vi "main_PC.vi"() -> ()   [LabVIEW 2017]
panel:
  in  "Tab Control":enum32{"Page 1", "Page 2"}(tab)
  in  "Menu Ring":u16(ring) items=["OFF", "Automatic", "Manual"]
  out "Waveform Chart":T1(graph) caption="Response Chart"
  in  "Pause Button":bool
  in  "Reset Chart":bool
  in  "Save as Excel":bool
  in  "Save as image":bool
  in  "Block Diagram":bool
  out "P":dbl
  out "Control Action":bool
  in  "Pressure setpoint":dbl=7.0 min=1.5 max=7.0
  in  "Comperssor":bool=TRUE
  in  "ON/OFF":bool
  in  "Exit":bool
  out "NI1":tag caption="NI device"
  in  "P 2":dbl
  in  "Main board":bool
  # "Pressure Control Training System"
  # "( 1.5-7 ) bar"
  # "Pressure sensor Reading"
  # "bar"
  # "Block Diagram of \nthe Pressure Closed-loop Control System"
  # "ON/OFF"
  # "Automatic mode"
  # "Actuator ON/OFF"
  # "desired P"
  # "Controller\n(ON/OFF)"
  # "Actuator\n(Compressor)"
  # "System"
  # "Pressure diff."
  # "error signal"
  # "+"
  # "-"
  # "Control Action\n(0 - 1)"
  # "actual P"
  # "Pressure sensor"
  # "Block Diagram of \nthe Pressure Open-loop Control System"
  # "Actuator ON/OFF"
  # "Actuator\n(Compressor)"
  # "Pressure diff."
  # "System"
  # "Press"
  # "Bush Button"
  # "Control Action\n(0 - 1)"
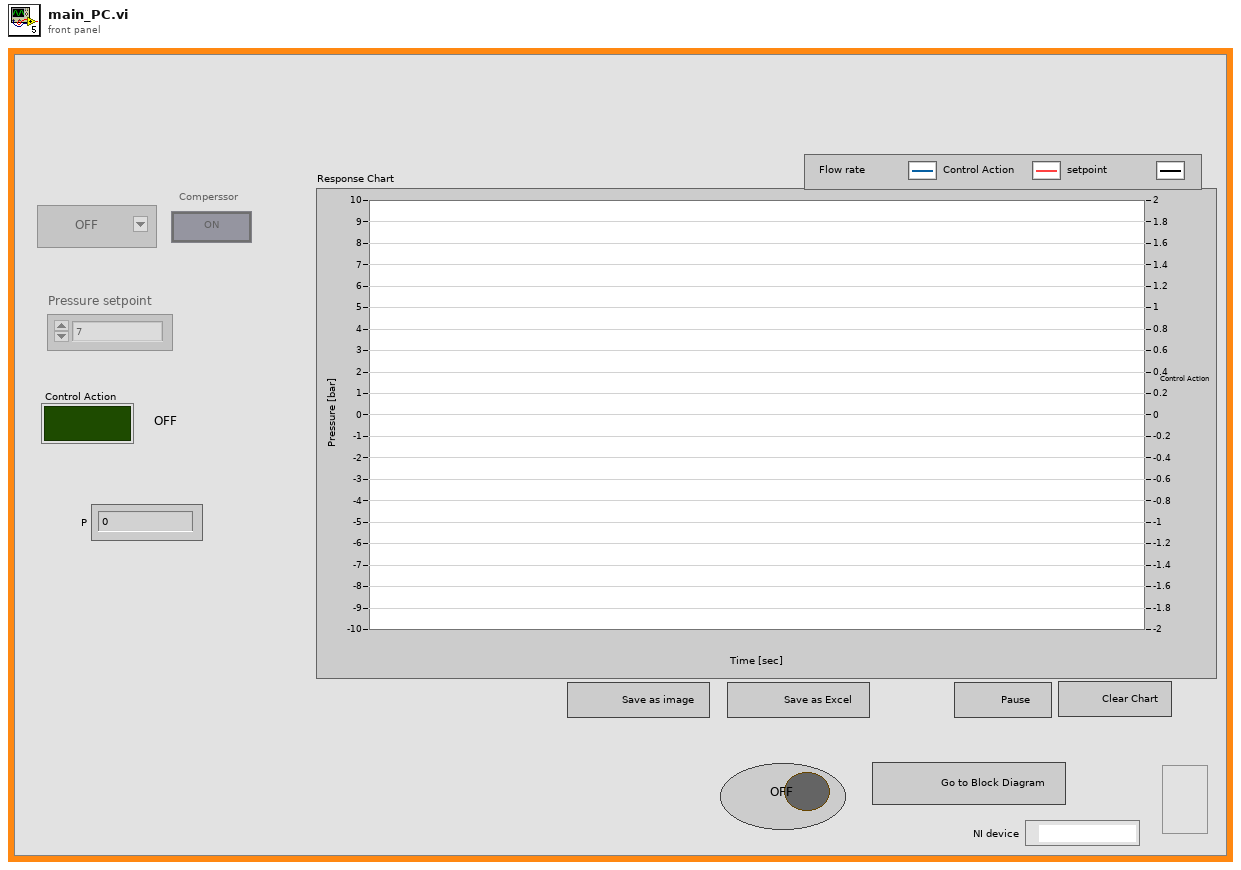
[diagram p1: front panel]
types:
  T1 = cluster{"Scalar":dbl, "f":dbl, "Flow rate setpoint":dbl}
  T2 = enum32{"Invalid", "Standard", "Closed", "Hidden", "Minimized", "Maximized"}
  T3 = enum8{"Enabled", "Disabled", "Disabled and Grayed Out"}
  T4 = cluster{"Scalar":dbl, "f":dbl, "Flow rate setpoint":dbl}[]
  T5 = cluster{"Scalar":dbl, i16, "Pressure setpoint":dbl}
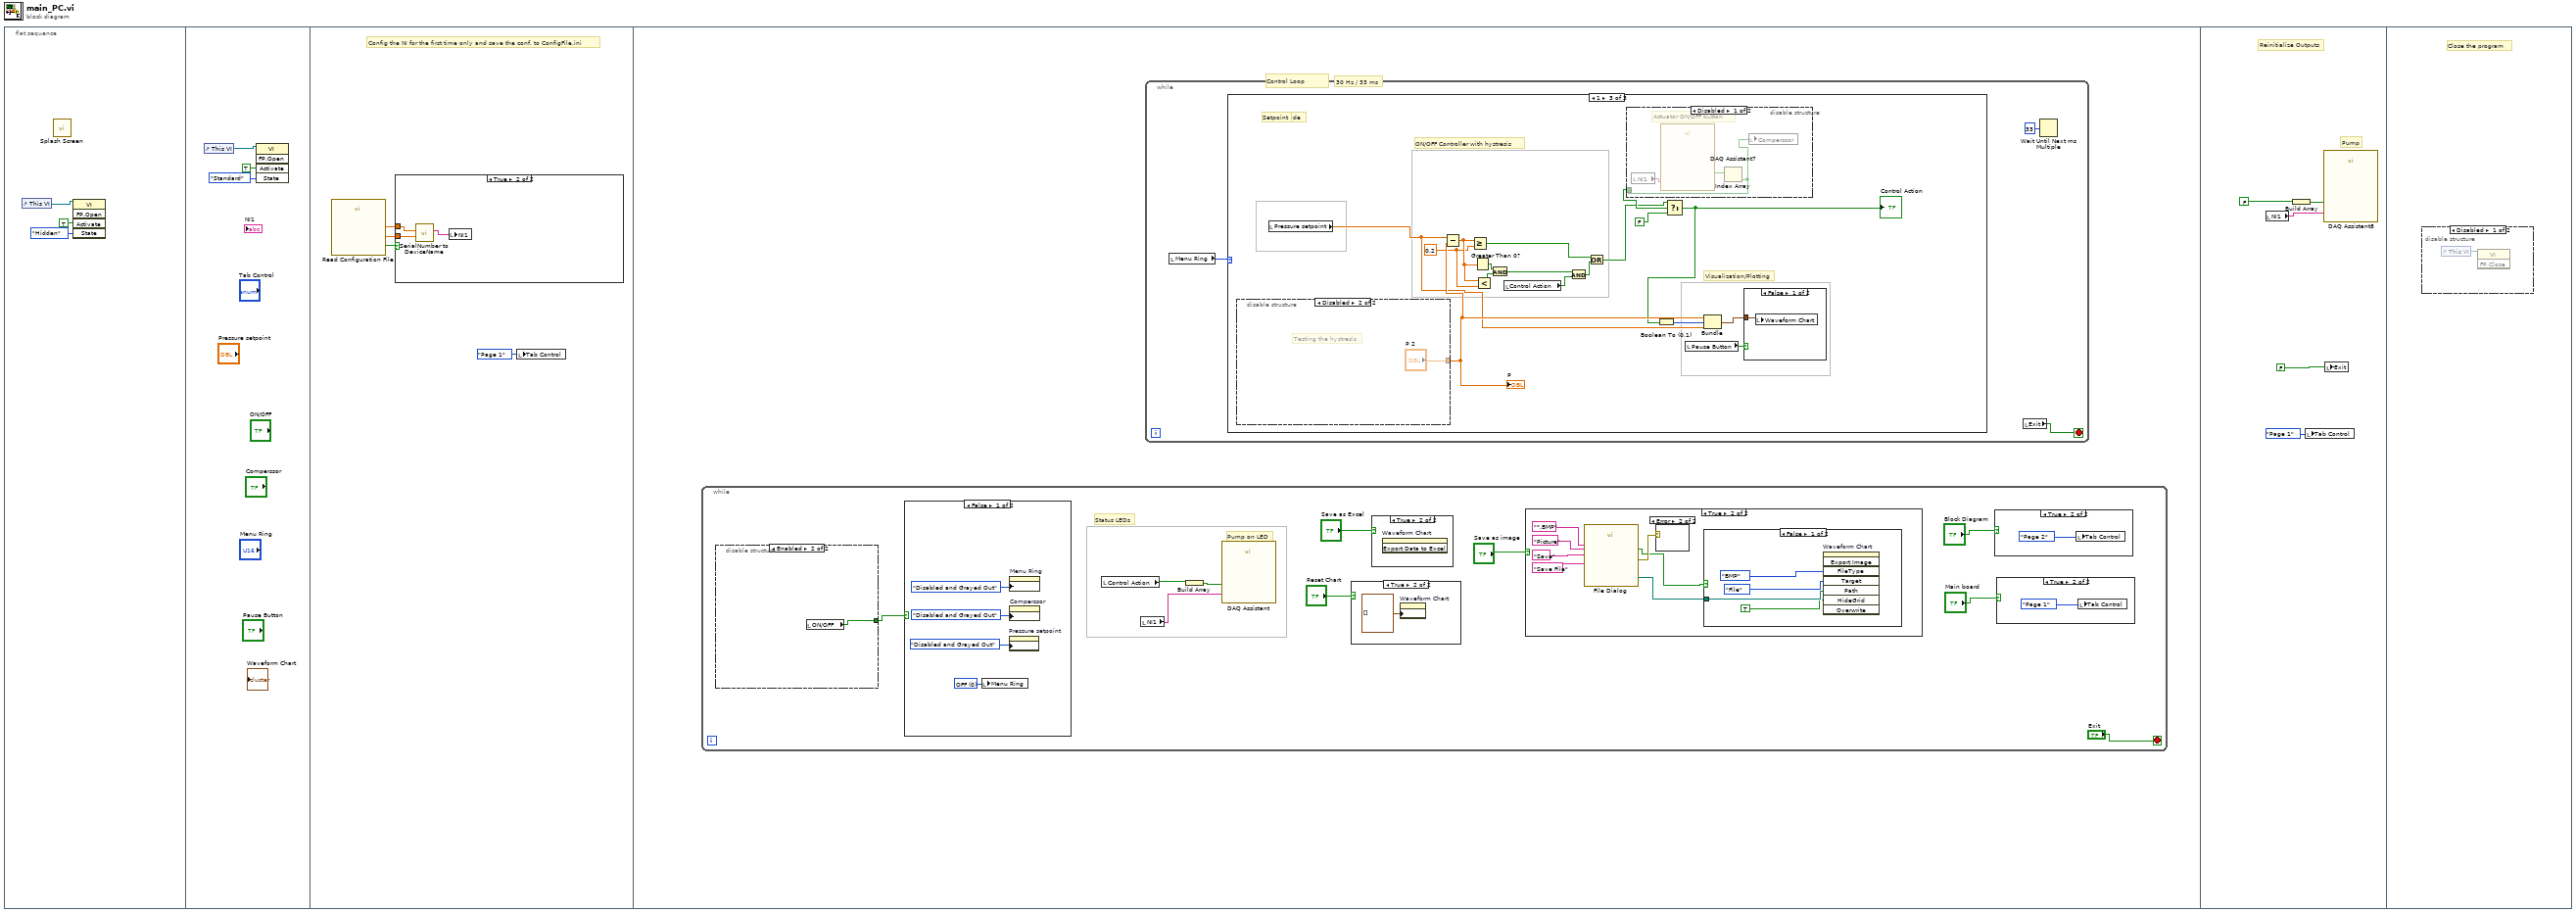
[diagram p0: block diagram]
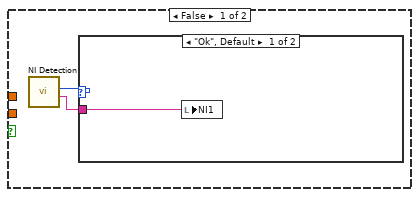
[diagram p2: hidden frame]
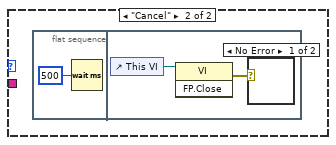
[diagram p3: hidden frame]
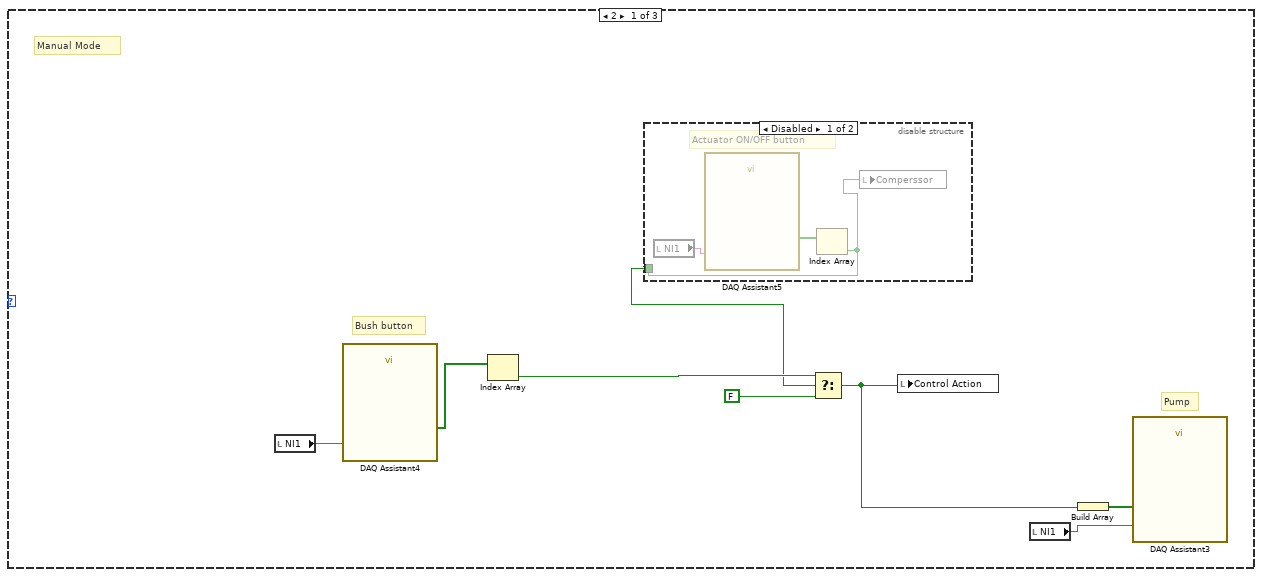
[diagram p5: hidden frame]
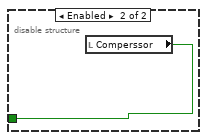
[diagram p6: hidden frame]
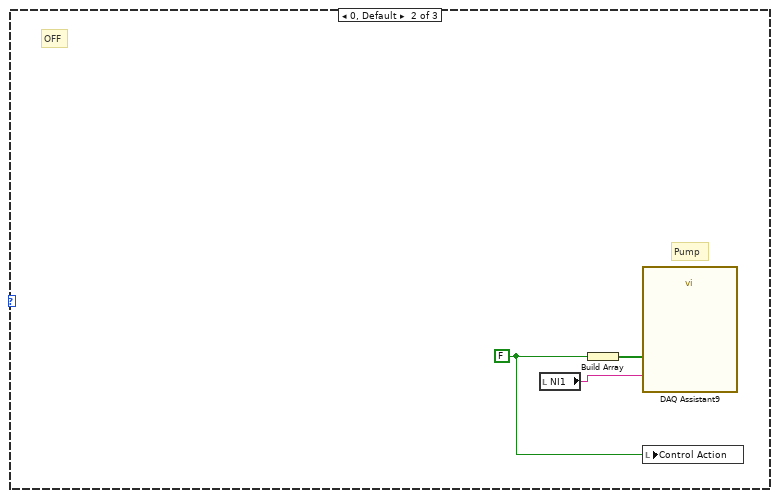
[diagram p7: hidden frame]
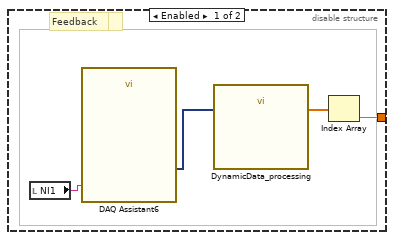
[diagram p8: hidden frame]
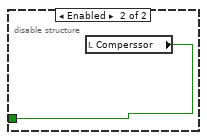
[diagram p9: hidden frame]
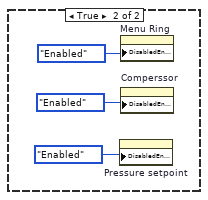
[diagram p11: hidden frame]
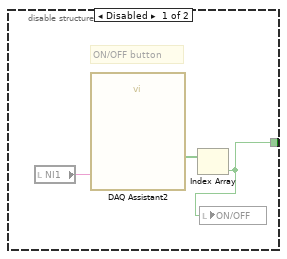
[diagram p12: hidden frame]
diagram:
  n1 = flat-sequence {
    frame #0 {
      n2 = control-ref of="This VI"() -> (w3:refnum<vi>)
      n3 = call "Splash Screen.vi"() -> ()  [unwired: 11 in, 1 out]
      n4 = invoke class="VI" method="FP.Open"(reference=w3, "Activate"=TRUE ("Activate?"), "State"=T2."Hidden") -> ()  [unwired: 2 in, 5 out]
    }
    frame #1 {
      n5 = control-ref of="This VI"() -> (w4:refnum<vi>)
      n6 = invoke class="VI" method="FP.Open"(reference=w4, "Activate"=TRUE ("Activate?"), "State"=T2."Standard") -> ()  [unwired: 2 in, 5 out]
    }
    frame #2 {
      # "Config the NI for the first time only and save the conf. to ConfigFile.ini"
      n7 = call "Read Configuration File.vi"() -> ("Serial Numbers Found"=w8:bool, "NI1"=w9:dbl, "NI2"=w10:dbl)  [unwired: 13 in]
      n8 = case shown="True" w8 {
        tunnel: w9 -> [_ w19]
        tunnel: w10 -> [_ w18]
        frame False {
          n9 = call "NI Detection.vi"() -> ("NI 1"=w11:tag, "Ok/Cancel"=w12:enum16{"Ok", "Cancel"})  [unwired: 8 in, 1 out]
          n10 = case shown="\"Ok\", Default" w12 {
            tunnel: w11 -> [w13 _]
            frame "Ok", Default {
              n11 = local write "NI1"(w13) -> ()
            }
            frame "Cancel" {
              n12 = flat-sequence {
                frame #0 {
                  n13 = Wait (ms)(milliseconds to wait=u32 500) -> ()  [unwired: 1 out]
                }
                frame #1 {
                  n14 = control-ref of="This VI"() -> (w16:refnum<vi>)
                  n15 = invoke class="VI" method="FP.Close"(reference=w16) -> (error out=w15:errorcluster)  [unwired: 2 in, 2 out]
                  n16 = case shown="No Error" w15 {
                    frame No Error {
                    }
                    frame Error {
                    }
                  }
                }
              }
            }
          }
        }
        frame True {
          n17 = call "SerialNumber to DeviceName.vi"("NI2 Serial Number"=w18, "NI1 Serial Number"=w19) -> ("NI1 Device Name"=w17:tag)  [unwired: 8 in, 1 out]
          n18 = local write "NI1"(w17) -> ()
        }
      }
      n19 = local write "Tab Control"(enum32{"Page 1", "Page 2"}."Page 1" ("Tab Control")) -> ()
    }
    frame #3 {
      # "30 Hz / 33 ms"
      # "Control Loop"
      n20 = while {
        stop <- "Exit" stop-if-true
        # "Pump on LED"
        # "Status LEDs"
        n21 = disable-structure shown="Enabled" {
          disable-tunnel: [w82 w85] -> w65
          frame Disabled {
            # "ON/OFF button"
            n22 = local read "NI1"() -> (w84:tag)
            n23 = call "DAQ Assistant2"("device name"=w84) -> ("data"=w83:bool[])  [unwired: 16 in, 2 out]
            n24 = Index Array(array=w83) -> (element=w82:bool)  [unwired: 1 in]
            n25 = local write "ON/OFF"(w82) -> ()
          }
          frame Enabled {
            n26 = local read "ON/OFF"() -> (w85:bool)
          }
        }
        n27 = case shown="False" w65 {
          frame False {
            w75 = u16 0 items=["OFF", "Automatic", "Manual"] ("Menu Ring")
            n28 = local write "Menu Ring"(w75) -> ()
            n29 = property on="Pressure setpoint" class="DigNum (strict)"("DisabledEnum"=T3."Disabled and Grayed Out" ("Disabled")) -> ()  [unwired: 2 in, 2 out]
            n30 = property on="Menu Ring" class="Ring (strict)"("DisabledEnum"=T3."Disabled and Grayed Out" ("Disabled")) -> ()  [unwired: 2 in, 2 out]
            n31 = property on="Comperssor" class="Bool (strict)"("DisabledEnum"=T3."Disabled and Grayed Out" ("Disabled")) -> ()  [unwired: 2 in, 2 out]
          }
          frame True {
            n32 = property on="Pressure setpoint" class="DigNum (strict)"("DisabledEnum"=T3."Enabled" ("Disabled")) -> ()  [unwired: 2 in, 2 out]
            n33 = property on="Menu Ring" class="Ring (strict)"("DisabledEnum"=T3."Enabled" ("Disabled")) -> ()  [unwired: 2 in, 2 out]
            n34 = property on="Comperssor" class="Bool (strict)"("DisabledEnum"=T3."Enabled" ("Disabled")) -> ()  [unwired: 2 in, 2 out]
          }
        }
        n35 = local read "Control Action"() -> (w67:bool)
        n36 = local read "NI1"() -> (w69:tag)
        n37 = Build Array(w67) -> (w68:bool[])
        n38 = call "DAQ Assistant"("data"=w68, "device name"=w69) -> ()  [unwired: 16 in, 2 out]
        n39 = case shown="True" "Reset Chart" {
          frame False {
          }
          frame True {
            n40 = property on="Waveform Chart" class="WFChart (strict)"("History Data"=T4 []) -> ()  [unwired: 2 in, 2 out]
          }
        }
        n41 = case shown="True" "Save as Excel" {
          frame False {
          }
          frame True {
            n42 = invoke on="Waveform Chart" class="WFChart (strict)" method="Export Data to Excel"() -> ()  [unwired: 3 in, 3 out]
          }
        }
        n43 = case shown="True" "Save as image" {
          frame False {
          }
          frame True {
            n44 = call "File Dialog"("prompt"="Save File", "button label"="Save", "pattern (all files)"="*.BMP", "pattern label"="Picture") -> ("selected path"=w87:path, "cancelled"=w86:bool, "error out"=w88:errorcluster)  [unwired: 8 in, 1 out]
            n45 = case shown="Error" w88 {
              frame No Error {
              }
              frame Error {
              }
            }
            n46 = case shown="False" w86 {
              tunnel: w87 -> [w94 _]
              frame False {
                n47 = invoke on="Waveform Chart" class="WFChart (strict)" method="Export Image"("FileType"=enum32{"BMP", "EPS", "EMF", "PICT"}."BMP" ("File Type"), "Target"=enum32{"File", "Clipboard"}."File", "Path"=w94, "HideGrid"=TRUE ("Hide Grid")) -> ()  [unwired: 4 in, 8 out]
              }
              frame True {
              }
            }
          }
        }
        n48 = case shown="True" "Block Diagram" {
          frame False {
          }
          frame True {
            n49 = local write "Tab Control"(enum32{"Page 1", "Page 2"}."Page 2" ("Tab Control")) -> ()
          }
        }
        n50 = case shown="True" "Main board" {
          frame False {
          }
          frame True {
            n51 = local write "Tab Control"(enum32{"Page 1", "Page 2"}."Page 1" ("Tab Control")) -> ()
          }
        }
      }
      n52 = while {
        stop <- w20 stop-if-true
        n53 = local read "Menu Ring"() -> (w21:u16)
        n54 = case shown="1" w21 {
          frame 2 {
            # "Pump"
            # "Manual Mode"
            # "Bush button"
            n55 = local read "NI1"() -> (w28:tag)
            n56 = call "DAQ Assistant4"("device name"=w28) -> ("data"=w27:bool[])  [unwired: 16 in, 2 out]
            n57 = Index Array(array=w27) -> (element=w30:bool)  [unwired: 1 in]
            n58 = disable-structure shown="Disabled" {
              disable-tunnel: [w32 w34] -> w29
              frame Disabled {
                # "Actuator ON/OFF button"
                n59 = local read "NI1"() -> (w31:tag)
                n60 = call "DAQ Assistant5"("device name"=w31) -> ("data"=w33:bool[])  [unwired: 16 in, 2 out]
                n61 = Index Array(array=w33) -> (element=w32:bool)  [unwired: 1 in]
                n62 = local write "Comperssor"(w32) -> ()
              }
              frame Enabled {
                n63 = local read "Comperssor"() -> (w34:bool)
              }
            }
            n64 = Select(t=w30, s=w29, f=FALSE) -> (s? t:f=w23:bool)
            n65 = local write "Control Action"(w23) -> ()
            n66 = local read "NI1"() -> (w24:tag)
            n67 = Build Array(w23) -> (w25:bool[])
            n68 = call "DAQ Assistant3"("data"=w25, "device name"=w24) -> ()  [unwired: 16 in, 2 out]
          }
          frame 0, Default {
            w35 = FALSE
            # "OFF"
            # "Pump"
            n69 = local read "NI1"() -> (w36:tag)
            n70 = Build Array(w35) -> (w37:bool[])
            n71 = call "DAQ Assistant9"("data"=w37, "device name"=w36) -> ()  [unwired: 16 in, 2 out]
            n72 = local write "Control Action"(w35) -> ()
          }
          frame 1 {
            w45 = 0.2 ("y")
            # "AUTO mode"
            # "Setpoint"
            # "Visualization/Plotting"
            # "ON/OFF Controller with hystresis"
            n73 = disable-structure shown="Disabled" {
              disable-tunnel: [w55 "P 2"] -> w51
              frame Enabled {
                # "Feedback"
                # "Flow sensor"
                n74 = local read "NI1"() -> (w56:tag)
                n75 = call "DAQ Assistant6"("device name"=w56) -> ("data"=w58:dynamicdata)  [unwired: 16 in, 2 out]
                n76 = call "DynamicData_processing.vi"("data"=w58) -> ("DATA"=w57:dbl[])
                n77 = Index Array(array=w57) -> (element=w55:dbl)  [unwired: 1 in]
              }
              frame Disabled {
                # "Testing the hystresis"
              }
            }
            "P" <- w51
            n78 = local read "Pressure setpoint"() -> (w38:dbl)
            n79 = Subtract(x=w38, y=w51) -> (x-y=w46:dbl)
            n80 = Greater Or Equal?(x=w46, y=w45) -> (x >= y?=w49:bool)
            n81 = Greater Than 0?(x=w46) -> (x > 0?=w48:bool)
            n82 = Less?(x=w46, y=w45) -> (x < y?=w47:bool)
            n83 = And(x=w48, y=w47) -> (x .and. y?=w44:bool)
            n84 = local read "Control Action"() -> (w43:bool)
            n85 = And(x=w44, y=w43) -> (x .and. y?=w42:bool)
            n86 = Or(x=w49, y=w42) -> (x .or. y?=w41:bool)
            n87 = disable-structure shown="Disabled" {
              disable-tunnel: [w61 w63] -> w53
              frame Disabled {
                # "Actuator ON/OFF button"
                n88 = local read "NI1"() -> (w60:tag)
                n89 = call "DAQ Assistant7"("device name"=w60) -> ("data"=w62:bool[])  [unwired: 16 in, 2 out]
                n90 = Index Array(array=w62) -> (element=w61:bool)  [unwired: 1 in]
                n91 = local write "Comperssor"(w61) -> ()
              }
              frame Enabled {
                n92 = local read "Comperssor"() -> (w63:bool)
              }
            }
            n93 = Select(t=w41, s=w53, f=FALSE) -> (s? t:f=w39:bool)
            "Control Action" <- w39
            n94 = Boolean To (0,1)(Boolean=w39) -> (0, 1=w40:i16)
            n95 = local read "Pause Button"() -> (w52:bool)
            n96 = Bundle("Scalar"=w51, w40, "Pressure setpoint"=w38) -> (w54:T5)  [unwired: 1 in]
            n97 = case shown="False" w52 {
              tunnel: w54 -> [w64 _]
              frame False {
                n98 = local write "Waveform Chart"(w64) -> ()
              }
              frame True {
              }
            }
          }
        }
        n99 = local read "Exit"() -> (w20:bool)
        n100 = Wait Until Next ms Multiple(millisecond multiple=u32 33) -> ()  [unwired: 1 out]
      }
    }
    frame #4 {
      # "Pump"
      # "Reinitialize Outputs"
      n101 = local read "NI1"() -> (w102:tag)
      n102 = Build Array(FALSE) -> (w101:bool[])
      n103 = local write "Tab Control"(enum32{"Page 1", "Page 2"}."Page 1" ("Tab Control")) -> ()
      n104 = call "DAQ Assistant8"("data"=w101, "device name"=w102) -> ()  [unwired: 16 in, 2 out]
      n105 = local write "Exit"(FALSE ("Exit")) -> ()
    }
    frame #5 {
      # "Close the program"
      n106 = disable-structure shown="Disabled" {
        frame Disabled {
          n107 = control-ref of="This VI"() -> (w105:refnum<vi>)
          n108 = invoke class="VI" method="FP.Close"(reference=w105) -> ()  [unwired: 2 in, 3 out]
        }
        frame Enabled {
        }
      }
    }
  }
